vi "Write Allow Undefinded Values.vi"(5 "Allow Undefinded Values":bool, 9 "Combobox in":refnum<class "Combobox.lvclass">) -> (3 "Combobox out":refnum<class "Combobox.lvclass">)   [LabVIEW 2014, in "Raspberry Pi Compatible Compiler for LabVIEW.lvlib" / "Combobox.lvclass"]
uses:
  Combobox.lvclass
  Combobox.lvclass/Combobox.ctl
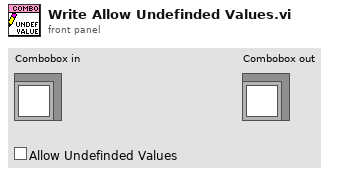
[diagram p1: front panel]
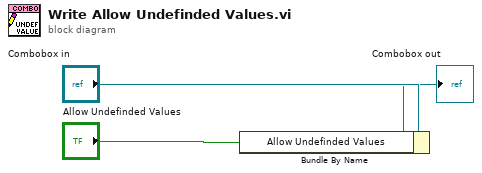
[diagram p0: block diagram]
diagram:
  n1 = Bundle By Name(cluster="Combobox in", "Allow Undefinded Values"="Allow Undefinded Values") -> (→"Combobox out":refnum<class "Combobox.lvclass">)
